vi "SC TCP Connect.vi"(6 "timeout ms (10000)":i32=10000, 8 "error in (no error)":errorcluster, 10 "port":u16, 11 "Server IP Address":string) -> (0 "error out":errorcluster, 2 "Connected":bool, 3 "TCP Network Connection out":refnum<k5>)   [LabVIEW 2018]
panel:
  out "data":string
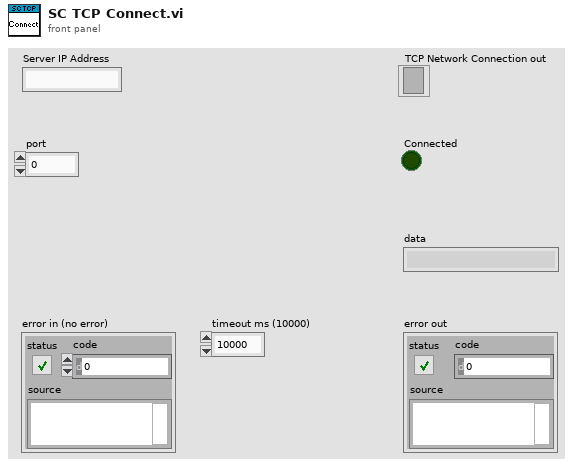
[diagram p1: front panel]
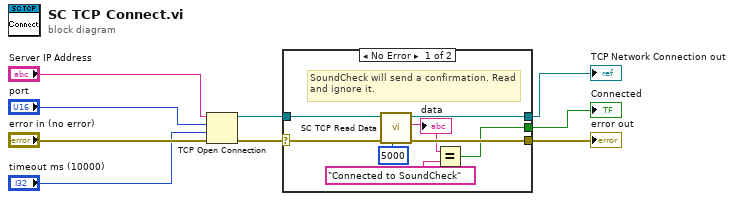
[diagram p0: block diagram]
diagram:
  n1 = TCP Open Connection(address="Server IP Address", remote port or service name="port", timeout ms (60000)="timeout ms (10000)", error in (no error)="error in (no error)") -> (connection ID=w8:refnum<k5>, error out=w4:errorcluster)  [unwired: 1 in]
  n2 = case shown="No Error" w4 {
    selector: w4 -> [w16 w18]
    tunnel: w8 -> [w17 w19]
    tunnel: [w10 _] -> w5
    tunnel: [w14 w18] -> w7
    tunnel: [w13 w19] -> w9
    frame No Error {
      # "SoundCheck will send a confirmation. Read and ignore it."
      n3 = call "SC TCP Read Data.vi"("timeout ms (25000)"=5000, "error in"=w16, "TCP  Connection in"=w17) -> ("error out"=w14:errorcluster, "data"=w12:string, "TCP  Connection out"=w13:refnum<k5>)  [unwired: 6 in]
      "data" <- w12
      n4 = Equal?(x=w12, y="Connected to SoundCheck") -> (x = y?=w10:bool)
    }
    frame Error {
    }
  }
  "TCP Network Connection out" <- w9
  "error out" <- w7
  "Connected" <- w5
